vi "Robot Global Data.vi"() -> ()   [LabVIEW 2015]
doc: "This global VI can contain as many global variables as you need. Place a control on the panel, give it a good name. To read or write to it from a VI, drag the icon to the diagram of that VI. You can also drag from the project. Click on the node to change which global you access. You shouldn't have multiple locations writing to a global or it will cause a race-condition."
uses:
  <vilib>/Rock Robotics/WPI/Camera/WPI_CameraImageSize.ctl
  <vilib>/Rock Robotics/WPI/DriverStation/WPI_DriverStationRobotMode2.ctl
  Drive/Drive States.ctl
panel:
  in  "Drive State":T1=enum."Start Throttle"
  in  "Reverse Drive":bool
  in  "Right Drivetrain":dbl
  in  "Left Drivetrain":dbl
  in  "LED toggle rate (ms)":u32=20
  in  "Right Joystick 2 X":dbl
  in  "Left Joystick 2 X":dbl
  in  "Right Joystick 2 Y":dbl
  in  "Left Joystick 2 Y":dbl
  in  "Right Joystick X":dbl
  in  "Left Joystick X":dbl
  in  "Right Joystick Y":dbl
  in  "Left Joystick Y":dbl
  in  "Robot Mode":T2
  in  "image size":T3=enum."320x240"
  in  "Enable Vision":bool=TRUE
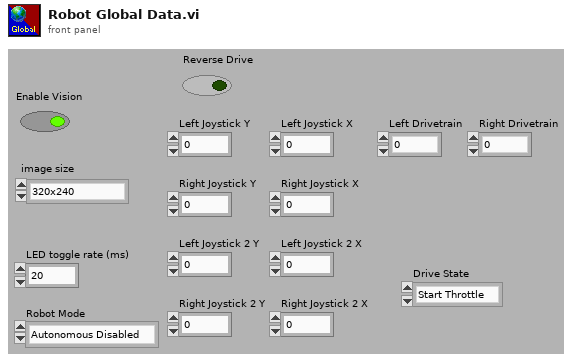
[diagram p1: front panel]
types:
  T1 = typedef "Drive States.ctl" = enum16{"Idle", "Teleop", "Start Rotate", "Do Rotate", "Stop Rotate", "Start Throttle", "Do Throttle", "Stop Throttle"}
  T2 = typedef "WPI_DriverStationRobotMode2.ctl" = enum16{"Autonomous Disabled", "Autonomous Enabled", "Teleop Disabled", "Teleop Enabled", "Disconnected", "Finish", "Test Disabled", "Test Enabled", "Emergency Stopped"}
  T3 = typedef "WPI_CameraImageSize.ctl" = enum16{"640x480", "320x240", "160x120", "Custom"}
diagram:
